vi "Read.vi"(8 "error in (no error)":errorcluster, 11 "Saving OO in":refnum<class "Saving OO.lvclass">) -> (0 "error out":errorcluster, 1 "Data(UTF8)":string[][](array[string]), 2 "Data(Text)":string[][](array[string]), 3 "Saving OO out":refnum<class "Saving OO.lvclass">)   [LabVIEW 2020, in "Saving OO.lvclass"]
uses:
  Saving OO.lvclass
  Saving OO.lvclass/Saving OO.ctl
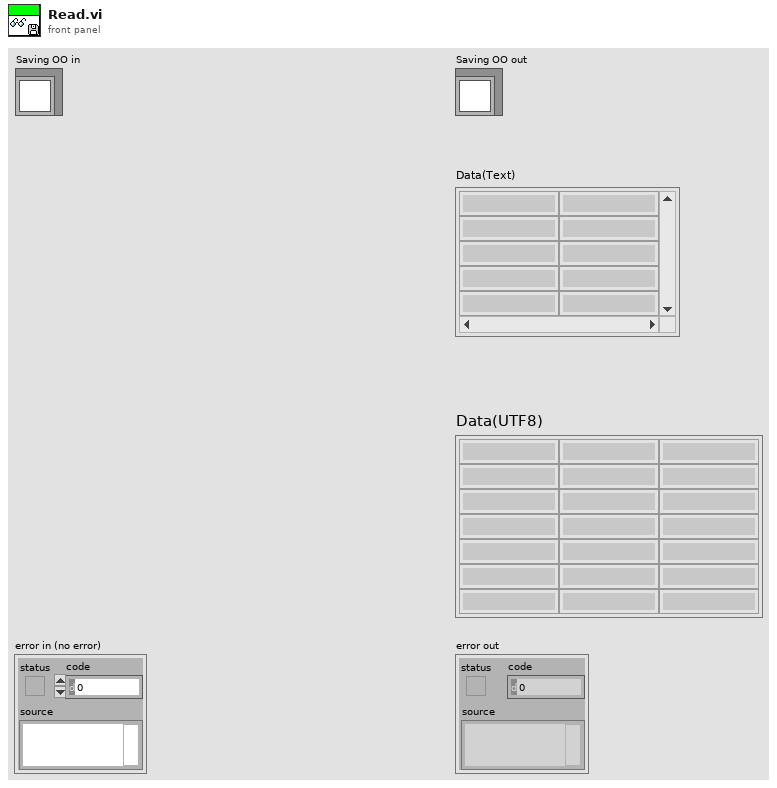
[diagram p1: front panel]
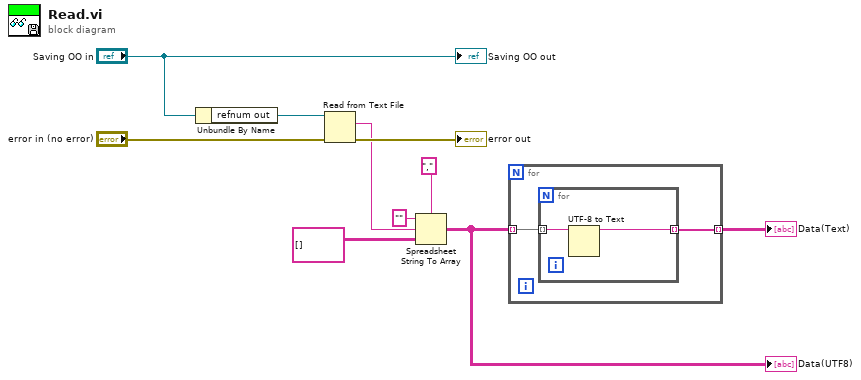
[diagram p0: block diagram]
diagram:
  n1 = Unbundle By Name("Saving OO in") -> ("refnum out"=w7:refnum<file>)
  n2 = Read from Text File(file (use dialog)=w7, error in="error in (no error)") -> (text=w4:string, error out=→"error out":errorcluster)  [unwired: 2 in, 2 out]
  n3 = Spreadsheet String To Array(delimiter (Tab)=",", format string="", spreadsheet string=w4, array type (2D Dbl)=string[][] []) -> (array=w2:string[][])
  "Data(UTF8)" <- w2
  n4 = for {
    tunnel: w2 -> [w12] mode=indexing
    tunnel: [w11] -> w1 mode=indexing
    n5 = for {
      tunnel: w12 -> [w14] mode=indexing
      tunnel: [w13] -> w11 mode=indexing
      n6 = UTF-8 to Text(11:w14) -> (3:w13:string)  [unwired: 2 in, 1 out]
    }
  }
  "Data(Text)" <- w1
  "Saving OO out" <- "Saving OO in"
